vi "graph4_2.vi"(11 "replay":bool) -> (0 "y":dynamicdata(graph), 3 "x":dynamicdata(graph), 4 "size(s)":i32)   [LabVIEW 2015]
uses:
  G_SEN.vi
  G_LCM.vi
  <vilib>/Analysis/polynomials.llb/1D Polynomial Evaluation (DBL).vi
  G_ALL.vi
  <vilib>/Analysis/NI_AALPro.lvlib
panel:
  in  "y 2":dbl=3.9000000000000004 format="%#_13g"
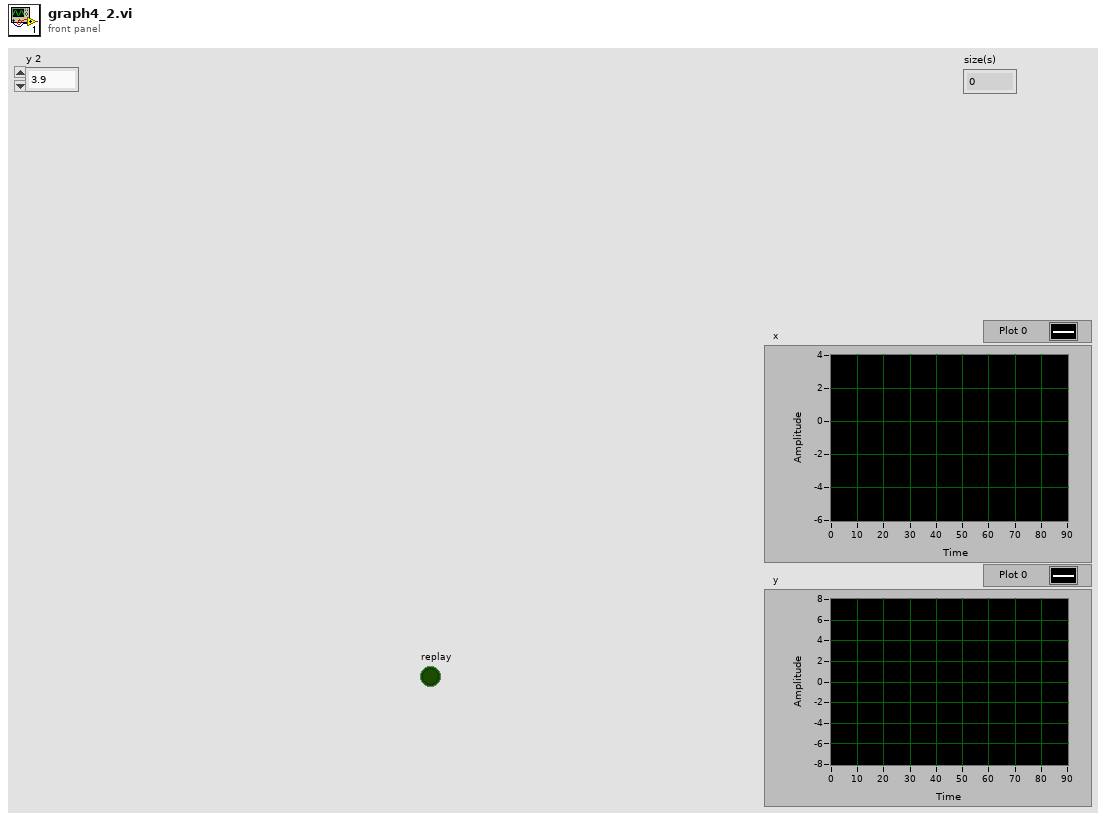
[diagram p1: front panel]
types:
  T1 = cluster{"Steer_input":dbl, "Steer_output":dbl, "VS_des":dbl, "VS_can":dbl, "heading":dbl, "auto":bool, "run":bool, "x":dbl, "y":dbl, "slam_y":dbl, "slam_x":dbl, "slam_heading":dbl}
  T2 = cluster{"C_Wheel base":dbl, "ratio_steer":dbl, "Overall width":dbl, "af":dbl, "turn radius":dbl, "eval":dbl, "ap":dbl, "an":dbl, "Vmax":dbl, "mu":dbl, "Vlast":dbl}
  T3 = cluster{"hash":i64, "sys time":i64, "stopline_exist":bool, "stopline_distance":dbl}
  T4 = cluster{"hash":i64, "sys time":i64, "n":i32, "Istone":cluster{"sys time":i64, "x":sgl, "y":sgl, "z":sgl}[], "Istone_dir":i64[]}
  T5 = cluster{"sys time":i64, "x":sgl, "y":sgl, "z":sgl}[]
  T6 = cluster{"sys time":i64, "x":sgl, "y":sgl, "z":sgl}
  T7 = cluster{"hash":i64, "sys time":i64, "size":i64, "x":dbl[], "y":dbl[]}
  T8 = cluster{"hash":i64, "sys time":i64, "time":dbl, "x":dbl, "y":dbl, "h":dbl, "numSV":i32, "postype":i32, "lag":i32, "hordev":dbl, "lat":dbl, "lon":dbl, "hgt":dbl, "map_idx":i32}
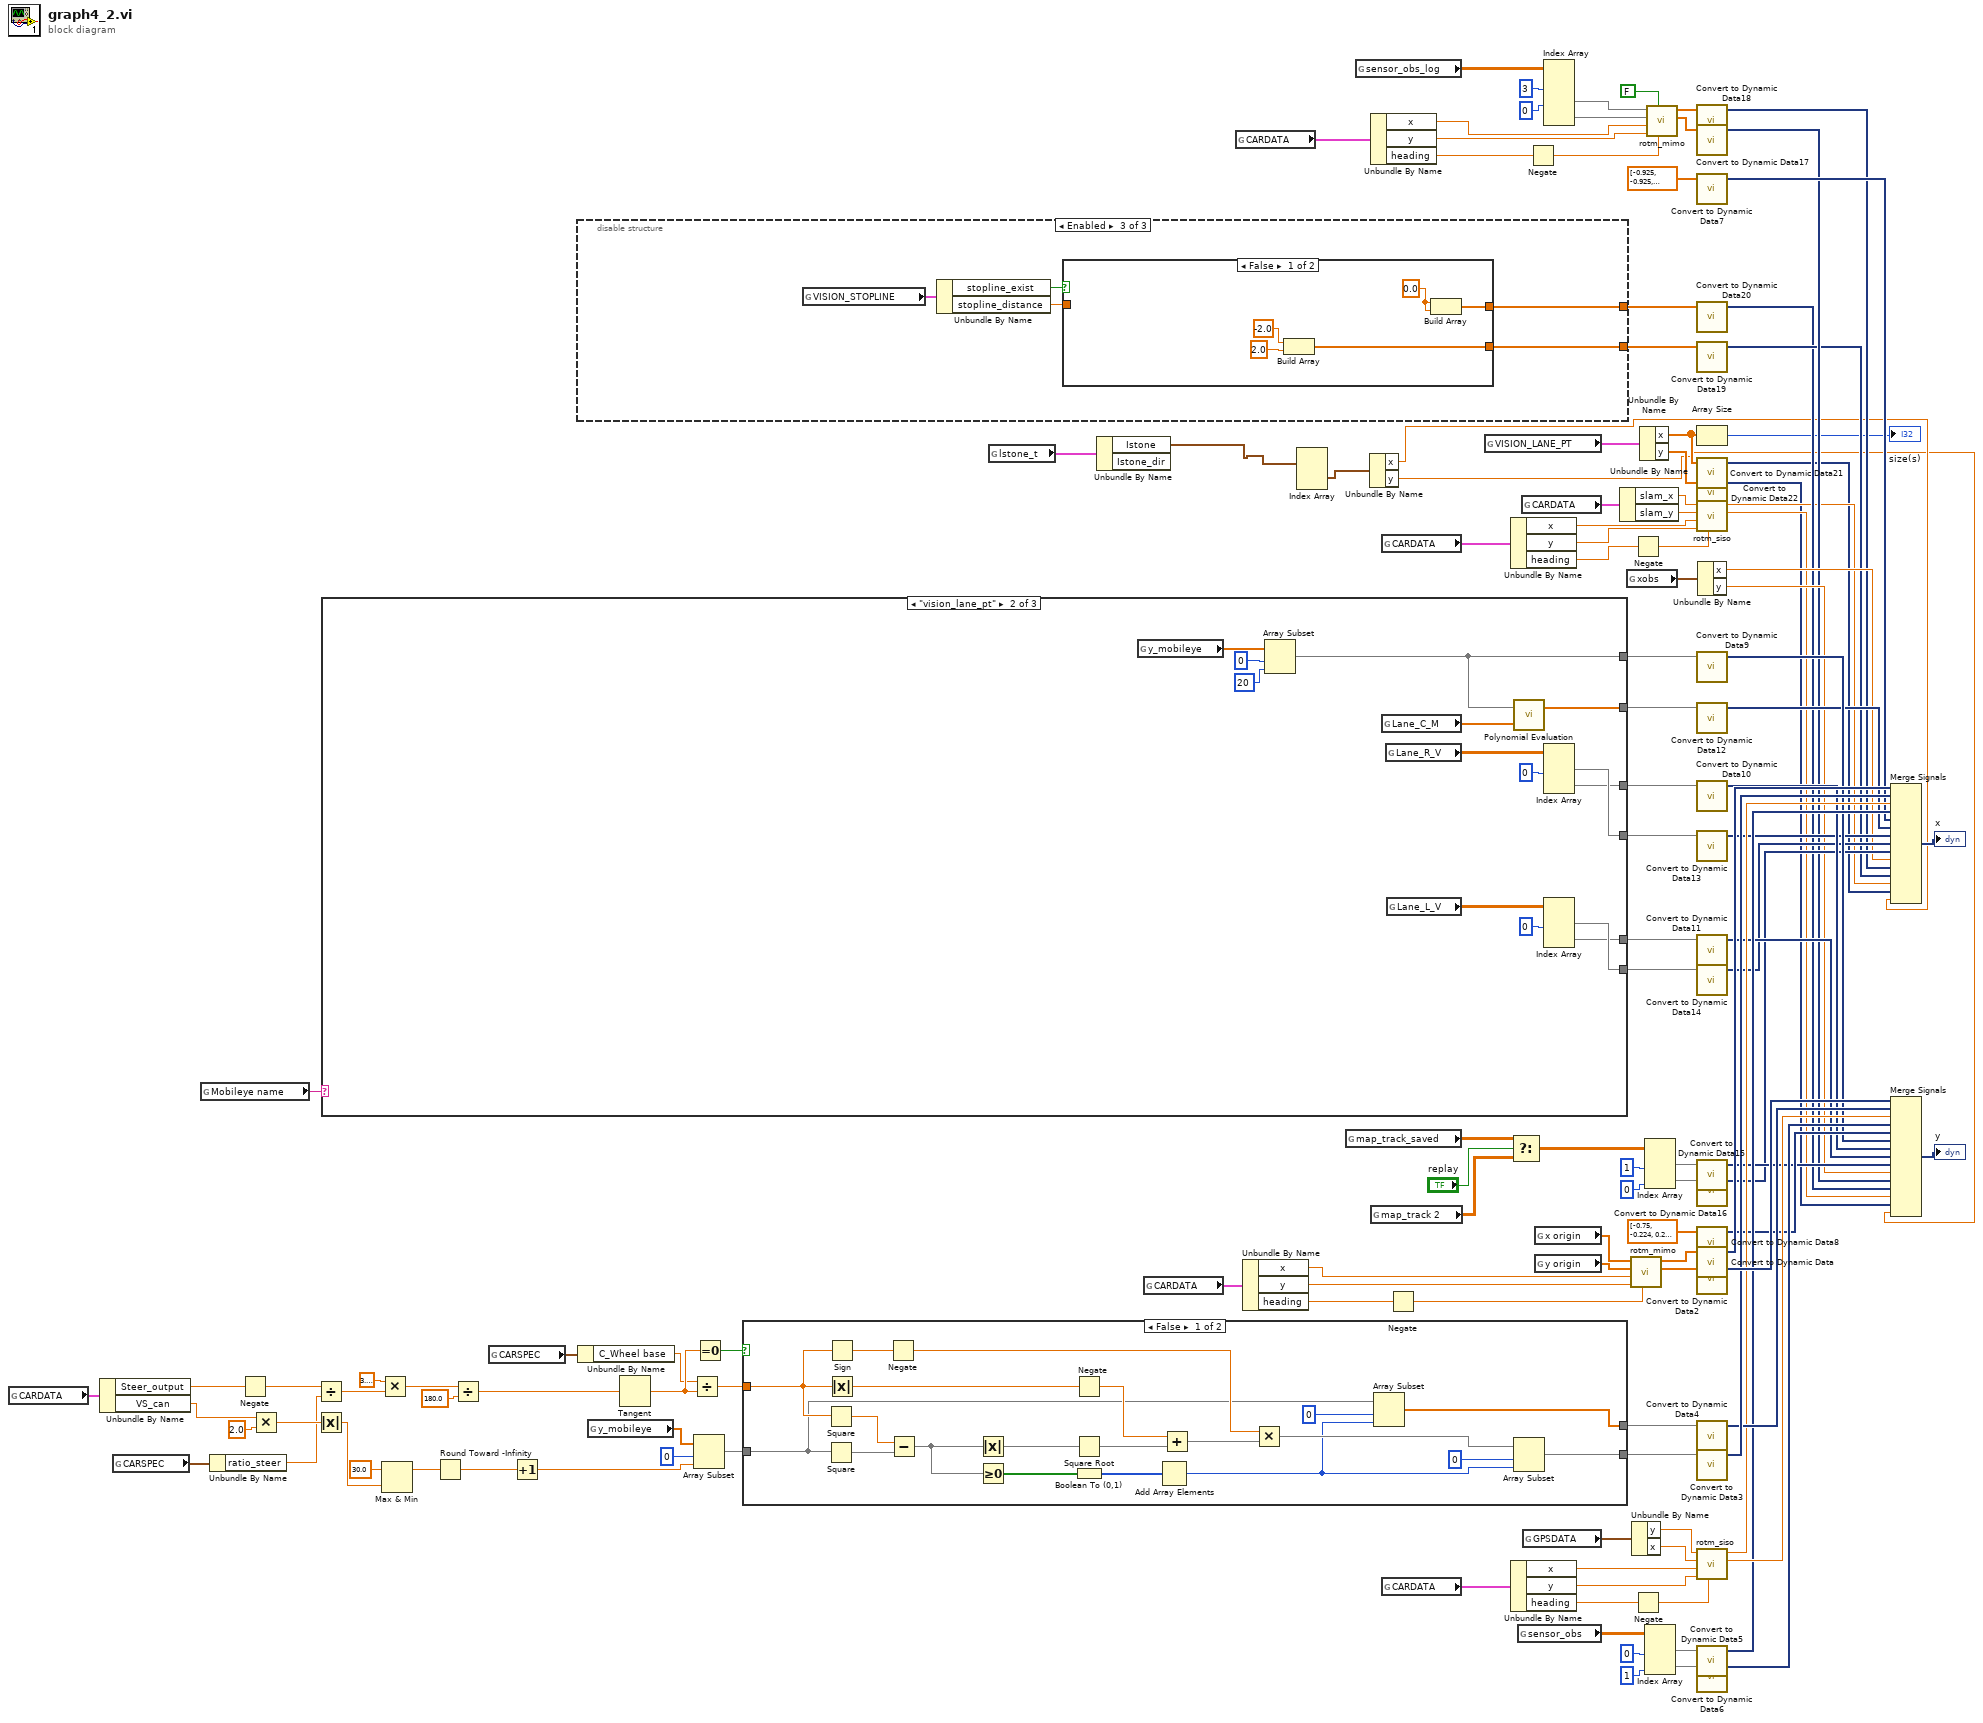
[diagram p0: block diagram]
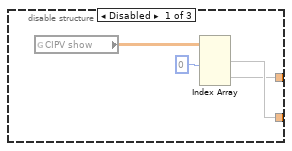
[diagram p2: hidden frame]
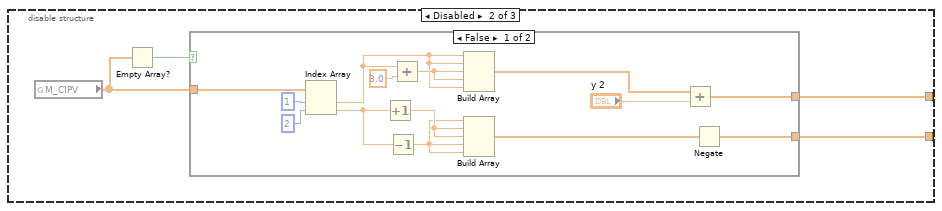
[diagram p3: hidden frame]
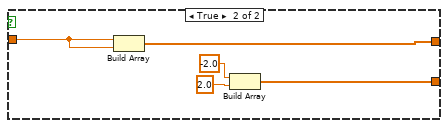
[diagram p5: hidden frame]
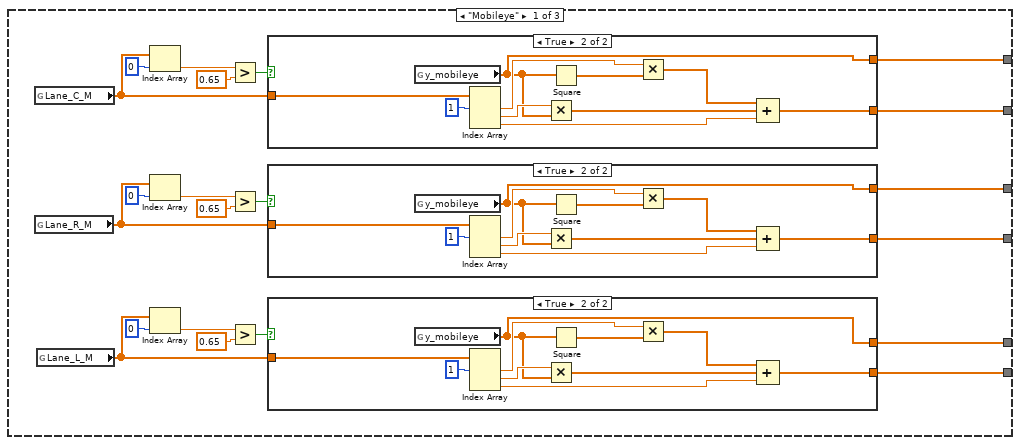
[diagram p6: hidden frame]
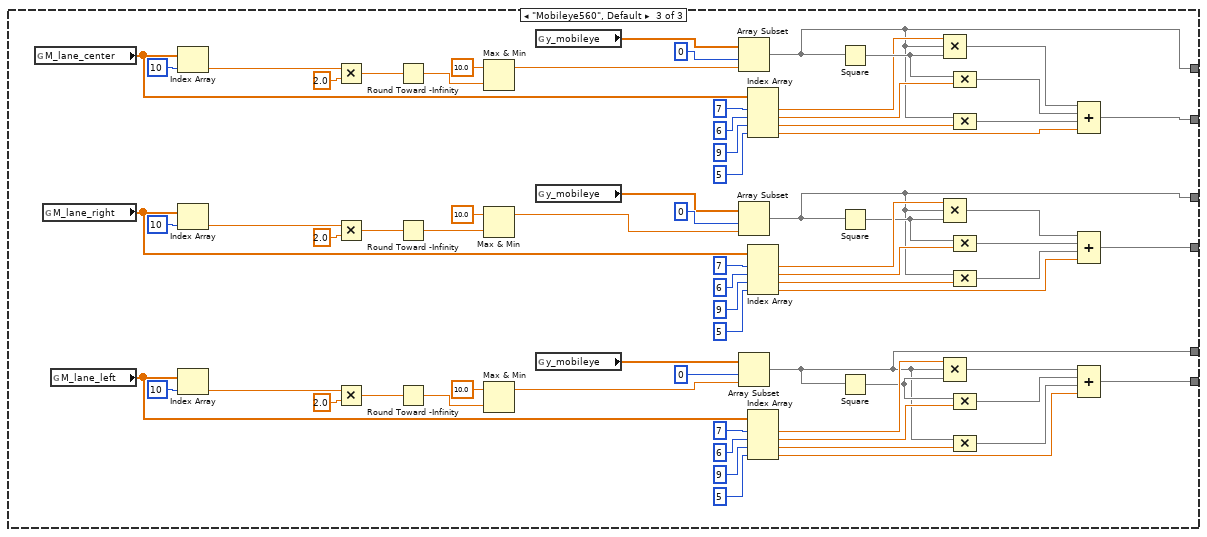
[diagram p10: hidden frame]
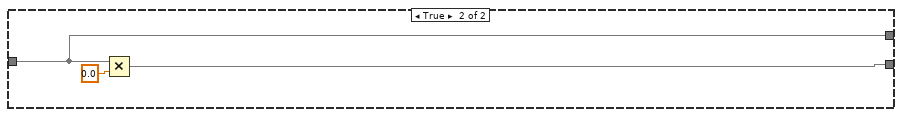
[diagram p11: hidden frame]
diagram:
  n1 = global read "G_ALL.vi" "CARDATA"() -> (w35:T1)
  n2 = Unbundle By Name(w35) -> ("Steer_output"=w80:dbl, "VS_can"=w107:dbl)
  n3 = global read "G_ALL.vi" "CARSPEC"() -> (w24:T2)
  n4 = global read "G_LCM.vi" "Mobileye name"() -> (w76:string)
  n5 = Unbundle By Name(w24) -> ("ratio_steer"=w23:dbl)
  n6 = Negate(x=w80) -> (-x=w79:dbl)
  n7 = Multiply(x=w107, y=2.0) -> (x*y=w112:dbl)
  n8 = Divide(x=w79, y=w23) -> (x/y=w122:dbl)
  n9 = Absolute Value(x=w112) -> (abs(x)=w113:dbl)
  n10 = case shown="\"vision_lane_pt\"" w76 {
    tunnel: [w146 w183 w201] -> w75
    tunnel: [w139 w188 w200] -> w73
    tunnel: [w132 w184 w199] -> w71
    tunnel: [w145 w195 w198] -> w69
    tunnel: [w138 w189 w197] -> w67
    tunnel: [w131 w185 w196] -> w65
    frame "Mobileye" {
      n11 = global read "G_SEN.vi" "Lane_C_M"() -> (w150:dbl[])
      n12 = global read "G_SEN.vi" "Lane_R_M"() -> (w141:dbl[])
      n13 = global read "G_SEN.vi" "Lane_L_M"() -> (w136:dbl[])
      n14 = Index Array(array=w150, index=0) -> (element=w148:dbl)
      n15 = Index Array(array=w141, index=0) -> (element=w143:dbl)
      n16 = Index Array(array=w136, index=0) -> (element=w134:dbl)
      n17 = Greater?(x=w148, y=0.65) -> (0:w149:bool)
      n18 = Greater?(x=w143, y=0.65) -> (0:w142:bool)
      n19 = Greater?(x=w134, y=0.65) -> (0:w135:bool)
      n20 = case shown="True" w149 {
        tunnel: w150 -> [_ w173]
        tunnel: [_ w174] -> w145
        tunnel: [_ w172] -> w146
        frame False {
        }
        frame True {
          n21 = global read "G_SEN.vi" "y_mobileye"() -> (w172:dbl[])
          n22 = Index Array(array=w173, index #1=1 ("index")) -> (element #1=w179:dbl, element #2=w178:dbl, element #3=w175:dbl)  [unwired: 2 in]
          n23 = Multiply(x=w178, y=w172) -> (x*y=w176:dbl[])
          n24 = Square(x=w172) -> (x^2=w180:dbl[])
          n25 = Multiply(x=w179, y=w180) -> (x*y=w177:dbl[])
          n26 = Compound Arithmetic op=ADD(w177, w176, w175) -> (w174:dbl[])
        }
      }
      n27 = case shown="True" w142 {
        tunnel: w141 -> [_ w163]
        tunnel: [_ w164] -> w138
        tunnel: [_ w162] -> w139
        frame False {
        }
        frame True {
          n28 = global read "G_SEN.vi" "y_mobileye"() -> (w162:dbl[])
          n29 = Index Array(array=w163, index #1=1 ("index")) -> (element #1=w169:dbl, element #2=w168:dbl, element #3=w165:dbl)  [unwired: 2 in]
          n30 = Multiply(x=w168, y=w162) -> (x*y=w166:dbl[])
          n31 = Square(x=w162) -> (x^2=w170:dbl[])
          n32 = Multiply(x=w169, y=w170) -> (x*y=w167:dbl[])
          n33 = Compound Arithmetic op=ADD(w167, w166, w165) -> (w164:dbl[])
        }
      }
      n34 = case shown="True" w135 {
        tunnel: w136 -> [_ w153]
        tunnel: [_ w154] -> w131
        tunnel: [_ w152] -> w132
        frame False {
        }
        frame True {
          n35 = global read "G_SEN.vi" "y_mobileye"() -> (w152:dbl[])
          n36 = Index Array(array=w153, index #1=1 ("index")) -> (element #1=w159:dbl, element #2=w158:dbl, element #3=w155:dbl)  [unwired: 2 in]
          n37 = Multiply(x=w158, y=w152) -> (x*y=w156:dbl[])
          n38 = Square(x=w152) -> (x^2=w160:dbl[])
          n39 = Multiply(x=w159, y=w160) -> (x*y=w157:dbl[])
          n40 = Compound Arithmetic op=ADD(w157, w156, w155) -> (w154:dbl[])
        }
      }
    }
    frame "vision_lane_pt" {
      n41 = global read "G_SEN.vi" "y_mobileye"() -> (w194:dbl[])
      n42 = Array Subset(array=w194, index=0, length=20) -> (w183:dbl[])
      n43 = global read "G_SEN.vi" "Lane_C_M"() -> (w182:dbl[])
      n44 = global read "G_SEN.vi" "Lane_R_V"() -> (w191:dbl[][])
      n45 = global read "G_SEN.vi" "Lane_L_V"() -> (w186:dbl[][])
      n46 = call-poly <vilib>:"Polynomial Evaluation.vi"("P(x)"=w182, "A"=w183) -> ("P(A)"=w195:dbl[])  [unwired: 1 out]
      n47 = Index Array(array=w191, index (col) #1=0 ("disabled index (col)")) -> (element #1=w189:dbl[], element #2=w188:dbl[])  [unwired: 3 in]
      n48 = Index Array(array=w186, index (col) #1=0 ("disabled index (col)")) -> (element #1=w185:dbl[], element #2=w184:dbl[])  [unwired: 3 in]
    }
    frame "Mobileye560", Default {
      n49 = global read "G_SEN.vi" "M_lane_center"() -> (w208:dbl[])
      n50 = global read "G_SEN.vi" "M_lane_right"() -> (w207:dbl[])
      n51 = global read "G_SEN.vi" "M_lane_left"() -> (w206:dbl[])
      n52 = Index Array(array=w208, index=10) -> (element=w214:dbl)
      n53 = Index Array(array=w207, index=10) -> (element=w243:dbl)
      n54 = Index Array(array=w206, index=10) -> (element=w236:dbl)
      n55 = Multiply(x=w214, y=2.0) -> (x*y=w225:dbl)
      n56 = Multiply(x=w243, y=2.0) -> (x*y=w242:dbl)
      n57 = Multiply(x=w236, y=2.0) -> (x*y=w237:dbl)
      n58 = Round Toward -Infinity(1:w225) -> (0:w211:dbl)
      n59 = Round Toward -Infinity(1:w242) -> (0:w234:dbl)
      n60 = Round Toward -Infinity(1:w237) -> (0:w230:dbl)
      n61 = Max & Min(x=10.0, y=w211) -> (max(x,y)=w228:dbl)  [unwired: 1 out]
      n62 = Max & Min(x=10.0, y=w234) -> (max(x,y)=w232:dbl)  [unwired: 1 out]
      n63 = Max & Min(x=10.0, y=w230) -> (max(x,y)=w229:dbl)  [unwired: 1 out]
      n64 = global read "G_SEN.vi" "y_mobileye"() -> (w202:dbl[])
      n65 = global read "G_SEN.vi" "y_mobileye"() -> (w204:dbl[])
      n66 = global read "G_SEN.vi" "y_mobileye"() -> (w203:dbl[])
      n67 = Array Subset(array=w202, index=0, length=w228) -> (w201:dbl[])
      n68 = Array Subset(array=w204, index=0, length=w232) -> (w200:dbl[])
      n69 = Array Subset(array=w203, index=0, length=w229) -> (w199:dbl[])
      n70 = Index Array(array=w208, index #1=7 ("index"), index #2=6 ("index"), index #3=9 ("index"), index #4=5 ("index")) -> (element #1=w209:dbl, element #2=w222:dbl, element #3=w220:dbl, element #4=w227:dbl)
      n71 = Index Array(array=w207, index #1=7 ("index"), index #2=6 ("index"), index #3=9 ("index"), index #4=5 ("index")) -> (element #1=w266:dbl, element #2=w264:dbl, element #3=w262:dbl, element #4=w258:dbl)
      n72 = Index Array(array=w206, index #1=7 ("index"), index #2=6 ("index"), index #3=9 ("index"), index #4=5 ("index")) -> (element #1=w248:dbl, element #2=w250:dbl, element #3=w252:dbl, element #4=w256:dbl)
      n73 = Square(x=w201) -> (x^2=w216:dbl[])
      n74 = Square(x=w200) -> (x^2=w245:dbl[])
      n75 = Square(x=w199) -> (x^2=w246:dbl[])
      n76 = Compound Arithmetic op=MULTIPLY(w209, w201, w216) -> (w219:dbl[])
      n77 = Compound Arithmetic op=MULTIPLY(w266, w200, w245) -> (w261:dbl[])
      n78 = Compound Arithmetic op=MULTIPLY(w248, w199, w246) -> (w253:dbl[])
      n79 = Compound Arithmetic op=MULTIPLY(w216, w222) -> (w218:dbl[])
      n80 = Compound Arithmetic op=MULTIPLY(w201, w220) -> (w217:dbl[])
      n81 = Compound Arithmetic op=MULTIPLY(w245, w264) -> (w260:dbl[])
      n82 = Compound Arithmetic op=MULTIPLY(w200, w262) -> (w259:dbl[])
      n83 = Compound Arithmetic op=MULTIPLY(w246, w250) -> (w254:dbl[])
      n84 = Compound Arithmetic op=MULTIPLY(w199, w252) -> (w255:dbl[])
      n85 = Compound Arithmetic op=ADD(w219, w218, w217, w227) -> (w198:dbl[])
      n86 = Compound Arithmetic op=ADD(w261, w260, w259, w258) -> (w197:dbl[])
      n87 = Compound Arithmetic op=ADD(w253, w254, w255, w256) -> (w196:dbl[])
    }
  }
  n88 = Multiply(x=3.141592653589793, y=w122) -> (x*y=w119:dbl)
  n89 = Max & Min(x=30.0, y=w113) -> (max(x,y)=w114:dbl)  [unwired: 1 out]
  n90 = Round Toward -Infinity(1:w114) -> (0:w109:dbl)
  n91 = Divide(x=w119, y=180.0) -> (x/y=w121:dbl)
  n92 = global read "G_ALL.vi" "CARSPEC"() -> (w25:T2)
  n93 = Increment(x=w109) -> (x+1=w111:dbl)
  n94 = disable-structure shown="Enabled" {
    disable-tunnel: [w269 w275 w291] -> w41
    disable-tunnel: [w268 w274 w290] -> w39
    frame Disabled {
      n95 = global read "G_SEN.vi" "CIPV show"() -> (w271:dbl[][])
      n96 = Index Array(array=w271, index (col) #1=0 ("disabled index (col)")) -> (element #1=w269:dbl[], element #2=w268:dbl[])  [unwired: 3 in]
    }
    frame Disabled {
      n97 = global read "G_SEN.vi" "M_CIPV"() -> (w272:dbl[])
      n98 = Empty Array?(array=w272) -> (empty?=w273:bool)
      n99 = case shown="False" w273 {
        tunnel: [w276 _] -> w275
        tunnel: [w279 _] -> w274
        tunnel: w272 -> [w281 _]
        frame False {
          n100 = Index Array(array=w281, index #1=1 ("index"), index #2=2 ("index")) -> (element #1=w282:dbl, element #2=w286:dbl)
          n101 = Increment(x=w286) -> (x+1=w287:dbl)
          n102 = Decrement(x=w286) -> (x-1=w285:dbl)
          n103 = Add(x=w282, y=3.0) -> (x+y=w283:dbl)
          n104 = Build Array(w282, w282, w283, w283, w282) -> (w280:dbl[])
          n105 = Build Array(w285, w287, w287, w285, w285) -> (w277:dbl[])
          n106 = Add(x=w280, y="y 2") -> (x+y=w279:dbl[])
          n107 = Negate(x=w277) -> (-x=w276:dbl[])
        }
        frame True {
        }
      }
    }
    frame Enabled {
      n108 = global read "G_LCM.vi" "VISION_STOPLINE"() -> (w292:T3)
      n109 = Unbundle By Name(w292) -> ("stopline_exist"=w293:bool, "stopline_distance"=w294:dbl)
      n110 = case shown="False" w293 {
        tunnel: w294 -> [_ w301]
        tunnel: [w297 w302] -> w291
        tunnel: [w296 w300] -> w290
        frame False {
          w295 = 0.0 ("element")
          n111 = Build Array(-2.0 ("element"), 2.0 ("element")) -> (w297:dbl[])
          n112 = Build Array(w295, w295) -> (w296:dbl[])
        }
        frame True {
          n113 = Build Array(w301, w301) -> (w300:dbl[])
          n114 = Build Array(-2.0 ("element"), 2.0 ("element")) -> (w302:dbl[])
        }
      }
    }
  }
  n115 = Unbundle By Name(w25) -> ("C_Wheel base"=w22:dbl)
  n116 = global read "G_SEN.vi" "y_mobileye"() -> (w106:dbl[])
  n117 = Tangent(1:w121) -> (0:w117:dbl)
  n118 = Divide(x=w22, y=w117) -> (x/y=w105:dbl)
  n119 = Array Subset(array=w106, index=0, length=w111) -> (w104:dbl[])
  n120 = Equal To 0?(x=w117) -> (x = 0?=w116:bool)
  n121 = case shown="False" w116 {
    tunnel: w105 -> [w320 _]
    tunnel: [w310 w325] -> w103
    tunnel: w104 -> [w308 w327]
    tunnel: [w306 w327] -> w101
    frame False {
      n122 = Square(x=w320) -> (x^2=w324:dbl)
      n123 = Square(x=w308) -> (x^2=w316:dbl[])
      n124 = Sign(1:w320) -> (0:w319:dbl)
      n125 = Absolute Value(x=w320) -> (abs(x)=w322:dbl)
      n126 = Negate(x=w319) -> (-x=w318:dbl)
      n127 = Subtract(x=w324, y=w316) -> (x-y=w314:dbl[])
      n128 = Absolute Value(x=w314) -> (abs(x)=w323:dbl[])
      n129 = Greater Or Equal To 0?(x=w314) -> (x >= 0?=w313:bool[])
      n130 = Negate(x=w322) -> (-x=w321:dbl)
      n131 = Square Root(x=w323) -> (sqrt(x)=w315:dbl[])
      n132 = Boolean To (0,1)(Boolean=w313) -> (0, 1=w312:i16[])
      n133 = Add Array Elements(numeric array=w312) -> (sum=w307:i16)
      n134 = Add(x=w321, y=w315) -> (x+y=w317:dbl[])
      n135 = Multiply(x=w318, y=w317) -> (x*y=w311:dbl[])
      n136 = Array Subset(array=w308, index=0, length=w307) -> (w306:dbl[])
      n137 = Array Subset(array=w311, index=0, length=w307) -> (w310:dbl[])
    }
    frame True {
      n138 = Multiply(x=w327, y=0.0) -> (x*y=w325:dbl[])
    }
  }
  n139 = global read "G_LCM.vi" "lstone_t"() -> (w5:T4)
  n140 = Unbundle By Name(w5) -> ("Istone"=w4:T5)  [unwired: 1 out]
  n141 = global read "G_ALL.vi" "CARDATA"() -> (w34:T1)
  n142 = global read "G_ALL.vi" "CARDATA"() -> (w32:T1)
  n143 = Unbundle By Name(w34) -> ("x"=w129:dbl, "y"=w128:dbl, "heading"=w130:dbl)
  n144 = Index Array(array=w4) -> (element #2=w3:T6)  [unwired: 3 in, 2 out]
  n145 = global read "G_ALL.vi" "map_track_saved"() -> (w28:dbl[][])
  n146 = global read "G_SEN.vi" "sensor_obs_log"() -> (w46:dbl[][])
  n147 = Unbundle By Name(w3) -> ("x"=w2:sgl, "y"=w1:sgl)
  n148 = Unbundle By Name(w32) -> ("x"=w51:dbl, "y"=w52:dbl, "heading"=w50:dbl)
  n149 = global read "G_ALL.vi" "map_track 2"() -> (w27:dbl[][])
  n150 = global read "G_ALL.vi" "CARDATA"() -> (w21:T1)
  n151 = global read "G_ALL.vi" "CARDATA"() -> (w33:T1)
  n152 = Negate(x=w130) -> (-x=w127:dbl)
  n153 = global read "G_LCM.vi" "VISION_LANE_PT"() -> (w12:T7)
  n154 = Unbundle By Name(w21) -> ("x"=w16:dbl, "y"=w17:dbl, "heading"=w15:dbl)
  n155 = Select(t=w28, s="replay", f=w27) -> (s? t:f=w36:dbl[][])
  n156 = Unbundle By Name(w33) -> ("x"=w98:dbl, "y"=w97:dbl, "heading"=w99:dbl)
  n157 = global read "G_SEN.vi" "sensor_obs"() -> (w89:dbl[][])
  n158 = global read "G_ALL.vi" "CARDATA"() -> (w6:T1)
  n159 = global read "G_ALL.vi" "GPSDATA"() -> (w31:T8)
  n160 = Negate(x=w50) -> (-x=w53:dbl)
  n161 = global read "G_ALL.vi" "x origin"() -> (w30:dbl[])
  n162 = global read "G_ALL.vi" "y origin"() -> (w29:dbl[])
  n163 = Index Array(array=w46, index (col) #1=3 ("disabled index (col)"), index (col) #2=0 ("disabled index (col)")) -> (element #2=w49:dbl[], element #3=w48:dbl[])  [unwired: 4 in, 1 out]
  n164 = Unbundle By Name(w6) -> ("slam_x"=w19:dbl, "slam_y"=w20:dbl)
  n165 = global read "G_ALL.vi" "xobs"() -> (w26:cluster{"idx":i32, "x":dbl, "y":dbl, "h":dbl})
  n166 = call "rotm_mimo.vi"("angle[rad]"=w127, "y0"=w128, "x0"=w129, "y"=w29, "x"=w30) -> ("Y"=w124:dbl[], "X"=w126:dbl[])  [unwired: 3 in, 2 out]
  n167 = Unbundle By Name(w31) -> ("y"=w95:dbl, "x"=w94:dbl)
  n168 = Negate(x=w15) -> (-x=w18:dbl)
  n169 = Negate(x=w99) -> (-x=w96:dbl)
  n170 = Unbundle By Name(w12) -> ("x"=w8:dbl[], "y"=w9:dbl[])
  n171 = Index Array(array=w36, index (col) #1=1 ("disabled index (col)"), index (col) #2=0 ("index (col)")) -> (element #1=w62:dbl[], element #2=w60:dbl[])  [unwired: 2 in]
  n172 = Index Array(array=w89, index (col) #1=0 ("disabled index (col)"), index (col) #2=1 ("index (col)")) -> (element #1=w88:dbl[], element #2=w86:dbl[])  [unwired: 2 in]
  n173 = call "rotm_mimo.vi"("angle[rad]"=w53, "reverse"=FALSE, "y0"=w52, "x0"=w51, "y"=w48, "x"=w49) -> ("Y"=w45:dbl[], "X"=w43:dbl[])  [unwired: 2 in, 2 out]
  n174 = call "Convert to Dynamic Data18"("Array"=w43) -> ("Dynamic Data Type"=w42:dynamicdata)  [unwired: 3 in]
  n175 = call "Convert to Dynamic Data17"("Array"=w45) -> ("Dynamic Data Type"=w44:dynamicdata)  [unwired: 3 in]
  n176 = call "Convert to Dynamic Data7"("Array"=dbl[] [-0.925, -0.925, -0.925, -0.6775, -0.6775, -0.925, -0.925, -0.925, -0.925, -0.6775, -0.6775, -0.925, -0.925, -0.925, 0.9025, 0.9025, 0.9025, 0.6775, 0.6775, 0.9025, 0.9025, 0.9025, 0.9025, 0.6775, 0.6775, 0.9025, 0.9025, 0.9025, -0.925] ("car_x")) -> ("Dynamic Data Type"=w84:dynamicdata)  [unwired: 3 in]
  n177 = call "Convert to Dynamic Data20"("Array"=w39) -> ("Dynamic Data Type"=w38:dynamicdata)  [unwired: 3 in]
  n178 = call "Convert to Dynamic Data19"("Array"=w41) -> ("Dynamic Data Type"=w40:dynamicdata)  [unwired: 3 in]
  n179 = Array Size(array=w8) -> (size(s)=→"size(s)":i32)
  n180 = call "Convert to Dynamic Data21"("Array"=w8) -> ("Dynamic Data Type"=w11:dynamicdata)  [unwired: 3 in]
  n181 = call "Convert to Dynamic Data22"("Array"=w9) -> ("Dynamic Data Type"=w10:dynamicdata)  [unwired: 3 in]
  n182 = call "rotm_siso.vi"("angle[rad]"=w18, "y0"=w17, "x0"=w16, "y"=w20, "x"=w19) -> ("y'"=w13:dbl, "x'"=w14:dbl)  [unwired: 5 in]
  n183 = call "Convert to Dynamic Data9"("Array"=w75) -> ("Dynamic Data Type"=w74:dynamicdata)  [unwired: 3 in]
  n184 = call "Convert to Dynamic Data12"("Array"=w69) -> ("Dynamic Data Type"=w68:dynamicdata)  [unwired: 3 in]
  n185 = call "Convert to Dynamic Data10"("Array"=w73) -> ("Dynamic Data Type"=w72:dynamicdata)  [unwired: 3 in]
  n186 = call "Convert to Dynamic Data13"("Array"=w67) -> ("Dynamic Data Type"=w66:dynamicdata)  [unwired: 3 in]
  n187 = call "Convert to Dynamic Data11"("Array"=w71) -> ("Dynamic Data Type"=w70:dynamicdata)  [unwired: 3 in]
  n188 = call "Convert to Dynamic Data14"("Array"=w65) -> ("Dynamic Data Type"=w64:dynamicdata)  [unwired: 3 in]
  n189 = call "Convert to Dynamic Data15"("Array"=w62) -> ("Dynamic Data Type"=w61:dynamicdata)  [unwired: 3 in]
  n190 = call "Convert to Dynamic Data16"("Array"=w60) -> ("Dynamic Data Type"=w59:dynamicdata)  [unwired: 3 in]
  n191 = call "Convert to Dynamic Data8"("Array"=dbl[] [-0.75, -0.224, 0.224, 0.224, -0.224, -0.224, 0.224, 2.415, 2.885, 2.885, 2.415, 2.415, 2.885, 3.5, 3.5, 2.885, 2.415, 2.415, 2.885, 2.885, 2.415, 0.224, -0.224, -0.224, 0.224, 0.224, -0.224, -0.75, -0.75] ("car_y")) -> ("Dynamic Data Type"=w83:dynamicdata)  [unwired: 3 in]
  n192 = call "Convert to Dynamic Data"("Array"=w126) -> ("Dynamic Data Type"=w125:dynamicdata)  [unwired: 3 in]
  n193 = call "Convert to Dynamic Data2"("Array"=w124) -> ("Dynamic Data Type"=w123:dynamicdata)  [unwired: 3 in]
  n194 = call "Convert to Dynamic Data4"("Array"=w101) -> ("Dynamic Data Type"=w100:dynamicdata)  [unwired: 3 in]
  n195 = call "Convert to Dynamic Data3"("Array"=w103) -> ("Dynamic Data Type"=w102:dynamicdata)  [unwired: 3 in]
  n196 = call "rotm_siso.vi"("angle[rad]"=w96, "y0"=w97, "x0"=w98, "y"=w94, "x"=w95) -> ("y'"=w92:dbl, "x'"=w93:dbl)  [unwired: 5 in]
  n197 = call "Convert to Dynamic Data5"("Array"=w88) -> ("Dynamic Data Type"=w87:dynamicdata)  [unwired: 3 in]
  n198 = call "Convert to Dynamic Data6"("Array"=w86) -> ("Dynamic Data Type"=w85:dynamicdata)  [unwired: 3 in]
  n199 = Unbundle By Name(w26) -> ("x"=w56:dbl, "y"=w57:dbl)
  n200 = Merge Signals(w125, w102, w93, w87, w84, w68, w66, w64, w59, w56, w42, w40, w14, w11, w2) -> (→"x":dynamicdata)
  n201 = Merge Signals(w123, w100, w92, w85, w83, w74, w72, w70, w61, w57, w44, w38, w13, w10, w1) -> (→"y":dynamicdata)
